vi "Insight_Laser_Load_Sensor.vi"(6 "Sensor File":string, 8 "error in (no error)":errorcluster, 11 "telnet connection":T1) -> (0 "error out":errorcluster, 2 "response data":string, 3 "telnet  connection out":T1)   [LabVIEW 2011]
doc: "Insight Photonic Solutions\n\nThis VI enables or disables Data Streaming when the laser is in Measurement Mode.\n\nver 1.0 - original release"
uses:
  Telnet Session.ctl
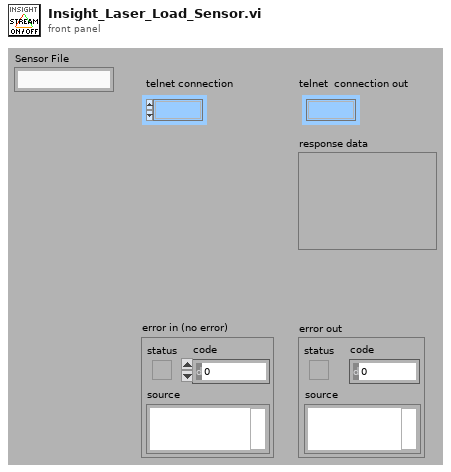
[diagram p1: front panel]
types:
  T1 = typedef "Telnet Session.ctl" = refnum<k1>
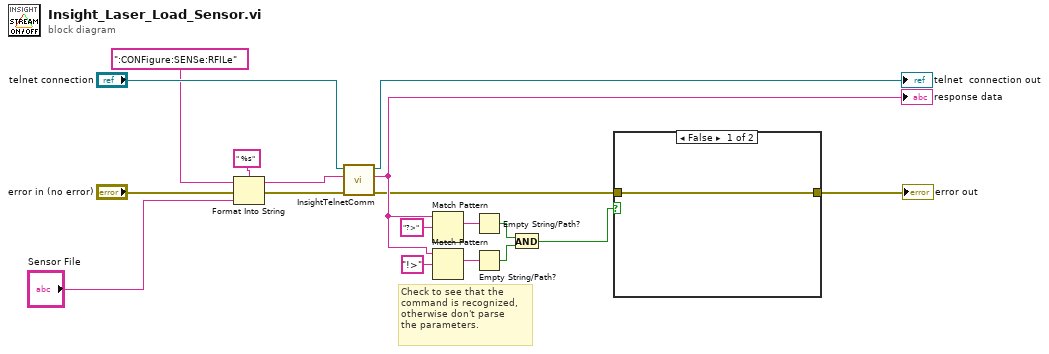
[diagram p0: block diagram]
diagram:
  # "Check to see that the \ncommand is recognized,\notherwise don't parse \nthe parameters."
  n1 = Format Into String(format string=" %s", initial string=":CONFigure:SENSe:RFILe" ("String"), error in="error in (no error)", "Sensor File") -> (resulting string=w16:string, error out=w17:errorcluster)
  n2 = call "InsightTelnetComm.vi"("error in"=w17, "write buffer (\"\")"=w16, "telnet connection"="telnet connection") -> ("error out"=w1:errorcluster, "response data"=w7:string, "telnet  connection out"=→"telnet  connection out":T1)  [unwired: 4 in]
  "response data" <- w7
  n3 = Match Pattern(string=w7, regular expression="?>") -> (match substring=w12:string)  [unwired: 1 in, 3 out]
  n4 = Match Pattern(string=w7, regular expression="!>") -> (match substring=w11:string)  [unwired: 1 in, 3 out]
  n5 = Empty String/Path?(string/path=w12) -> (empty?=w9:bool)
  n6 = Empty String/Path?(string/path=w11) -> (empty?=w8:bool)
  n7 = And(x=w9, y=w8) -> (x .and. y?=w3:bool)
  n8 = case shown="False" w3 {
    tunnel: [w19 w20] -> w2
    tunnel: w1 -> [w19 w20]
    frame False {
    }
    frame True {
    }
  }
  "error out" <- w2
